vi "LLProbe.vi"(11 "LinkedList":refnum<class "LinkedList.lvclass">) -> (2 "Value String":string, 3 "Boolean":bool)   [LabVIEW 2009, in "LinkedList.lvclass"]
uses:
  LinkedList.lvclass
panel:
  in  "Linked List":i32(listbox)
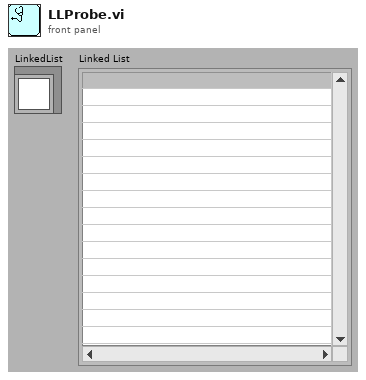
[diagram p1: front panel]
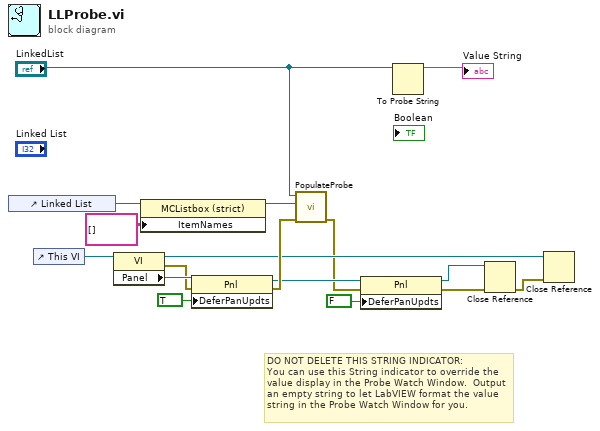
[diagram p0: block diagram]
diagram:
  # "DO NOT DELETE THIS STRING INDICATOR: \nYou can use this String indicator to override the value display in the Probe Watch Window.  Output an empty string to let LabVIEW format the value string in the Probe Watch Window for you."
  n1 = control-ref of="Linked List"() -> (w3:refnum<vi>)
  n2 = control-ref of="This VI"() -> (w16:refnum<vi>)
  n3 = property class="VI"(reference=w16) -> (reference out=w5:refnum<vi>, error out=w14:errorcluster, "Panel"=w15:refnum<vi>)  [unwired: 1 in]
  n4 = property class="MCListbox (strict)"(reference=w3, "ItemNames"=string[][] [] ("Item Names")) -> (reference out=w2:refnum<vi>)  [unwired: 1 in, 1 out]
  n5 = property class="Pnl"(reference=w15, error in=w14, "DeferPanUpdts"=TRUE ("Defer Panel Updates")) -> (reference out=w10:refnum<vi>, error out=w11:errorcluster)
  n6 = call "PopulateProbe.vi"("error in (no error)"=w11, "Multicolumn Listbox in"=w2, "LinkedList in"="LinkedList") -> ("error out"=w4:errorcluster)  [unwired: 6 in, 2 out]
  n7 = property class="Pnl"(reference=w10, error in=w4, "DeferPanUpdts"=FALSE ("Defer Panel Updates")) -> (reference out=w7:refnum<vi>, error out=w8:errorcluster)
  n8 = To Probe String(7:"LinkedList") -> (3:→"Value String":string)  [unwired: 2 in, 1 out]
  n9 = Close Reference(reference=w7, error in (no error)=w8) -> (error out=w6:errorcluster)
  n10 = Close Reference(reference=w5, error in (no error)=w6) -> ()  [unwired: 1 out]
